vi "sc5511a_reg_read.vi"(0 "deviceHandle":u32 format="%.0x", 2 "Register":T1(ring), 3 "Data In U64":u64 format="%.0x", 5 "error in":errorcluster) -> (14 "deviceHandle":u32 format="%.0x", 16 "Data Out":u64 format="%.0x", 19 "error out":errorcluster)   [LabVIEW 2010]
uses:
  sc5511a_rs232.dll
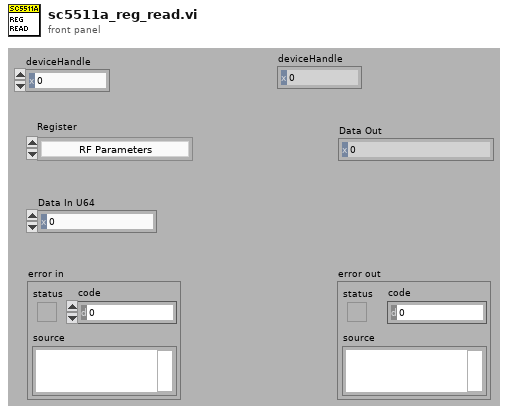
[diagram p1: front panel]
types:
  T1 = enum16{"RF Parameters", "Temperature", "Device Status", "Device Info", "List Buffer Read", "ALC Dac Value"}
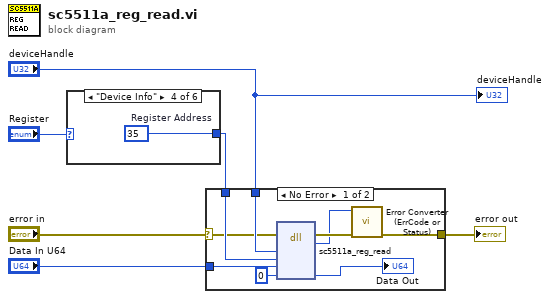
[diagram p0: block diagram]
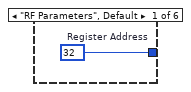
[diagram p2: hidden frame]
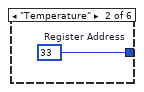
[diagram p3: hidden frame]
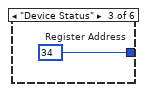
[diagram p4: hidden frame]
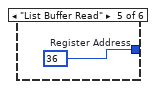
[diagram p5: hidden frame]
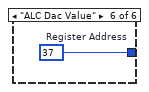
[diagram p6: hidden frame]
diagram:
  n1 = case shown="\"Device Info\"" "Register" {
    tunnel: [w7 w8 w9 w10 w11 w12] -> w3
    frame "RF Parameters", Default {
      w7 = u8 32  # Register Address
    }
    frame "Temperature" {
      w8 = u8 33  # Register Address
    }
    frame "Device Status" {
      w9 = u8 34  # Register Address
    }
    frame "Device Info" {
      w10 = u8 35  # Register Address
    }
    frame "List Buffer Read" {
      w11 = u8 36  # Register Address
    }
    frame "ALC Dac Value" {
      w12 = u8 37  # Register Address
    }
  }
  n2 = case shown="No Error" "error in" {
    selector: "error in" -> [w14 w22]
    tunnel: [w21 w22] -> w5
    tunnel: "deviceHandle" -> [w18 _]
    tunnel: w3 -> [w17 _]
    tunnel: "Data In U64" -> [w16 _]
    frame No Error {
      n3 = dll-call lib="I:/projects/falcon/sc5511a/development/software/api/rs232/comm32/labview/SignalCore/SC5511A-RS232/sc5511a_rs232.dll" fn="sc5511a_reg_read"(error in=w14, "deviceHandle"=w18, "Register"=w17, "Data In"=w16, "Data Out"=u64 0) -> (error out=w20:errorcluster, "return type"=w19:i32, "Data Out"=→"Data Out":u64)  [unwired: 5 in, 1 out]
      n4 = call "Error Converter (ErrCode or Status).vi"("error in (no error)"=w20, "error code"=w19) -> ("error out"=w21:errorcluster)  [unwired: 9 in]
    }
    frame Error {
    }
  }
  "error out" <- w5
  "deviceHandle" <- "deviceHandle"
